vi "lsl push sample d.vi"(8 "error in (no error)":errorcluster, 10 "data":dbl[](array[numeric]), 11 "outlet":u64) -> (0 "error out":errorcluster, 2 "function return":i32)   [LabVIEW 2019, in "Lab Streaming Layer.lvlib"]
doc: "extern LIBLSL_C_API int32_t lsl_push_sample_d(lsl_outlet out, const double *data);"
uses:
  Lab Streaming Layer.lvlib
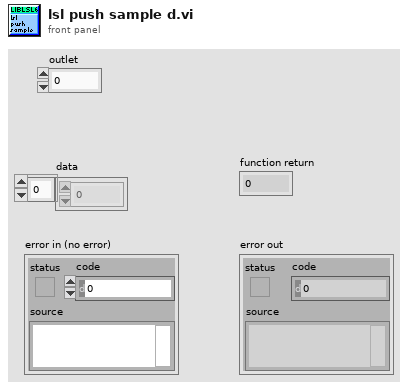
[diagram p1: front panel]
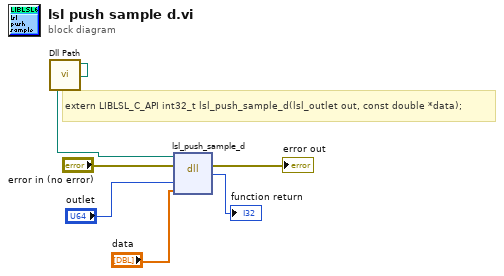
[diagram p0: block diagram]
diagram:
  # "extern LIBLSL_C_API int32_t lsl_push_sample_d(lsl_outlet out, const double *data);"
  n1 = call "Dll Path.vi"() -> ("Dll path"=w1:path)  [unwired: 11 in]
  n2 = dll-call lib="E:/LabStreamingLayer/liblsl-LabVIEW-master/liblsl-LabVIEW-master/lsl.dll" fn="lsl_push_sample_d"(path in=w1, error in="error in (no error)", "out"="outlet", "data"="data") -> (error out=→"error out":errorcluster, "return type"=→"function return":i32)  [unwired: 3 in, 1 out]
